vi "Constants.vi"() -> ()   [LabVIEW 2020, in "gRPC Server Shared.lvlib"]
doc: "Use this Global VI to access the GUIDs assigned to the page resources of the Custom Device."
uses:
  gRPC Server Shared.lvlib
panel:
  in  "Tab Control":enum32{"GUIDs", "Constants", "Properties"}(tab)
  in  "gRPC Server":string="b5bee5ca-c751-4925-818c-9ba70569fe08"
  in  "Compiled.Settings":string="Compiled.Settings"
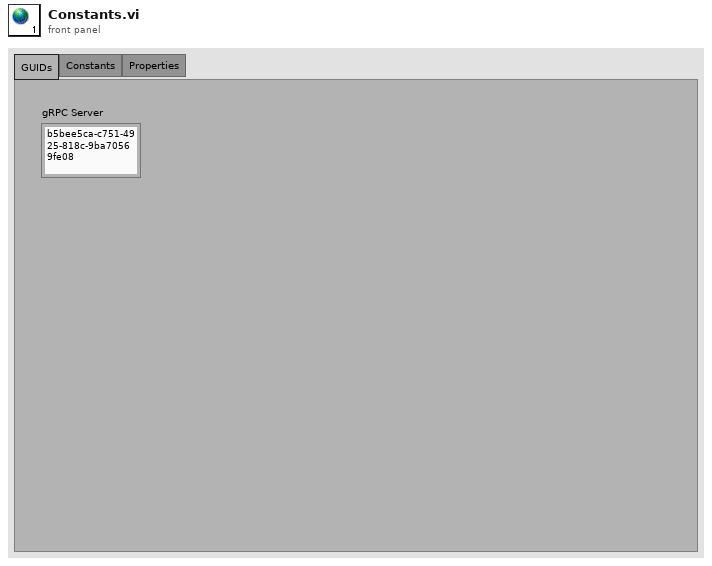
[diagram p1: front panel]
diagram:
